vi "Test Conversion.vi"() -> ()   [LabVIEW 2019]
uses:
  src/LV-Data/Typedefs/Map Variant--map.ctl
  <vilib>/numeric/Random Number (Range) U64.vi
  911225dc-c2b6-4d76-ae4e-277c5c34a072.vi
  d4c5f304-fa73-4c90-9b23-d6e558735612.vi
  816afb6b-e639-4658-a948-892f8dd4d78c.vi
  34a72b23-9838-41ec-bdf0-0bcc8987ef23.vi
  b954400e-7329-474c-b3d3-00700c715f51.vi
  6956be5f-2a95-4b1f-9b4a-a21892b67302.vi
  13e05168-3bdc-4092-8862-f966e558d68e.vi
  <vilib>/numeric/sub_Random U32.vi
  <vilib>/Utility/error.llb/Error Cluster From Error Code.vi
  <vilib>/addons/_JKI Toolkits/Caraya/classes/Assert/Assert Not Error.vi
  <vilib>/addons/_JKI Toolkits/Caraya/classes/Assert/Assert Equal Value_Variant.vi
  src/LV-Data/LV-Data.lvclass
  src/LV-Data/Typedefs/Dictionary--cluster.ctl
  67a28817-85e7-4f87-bc92-bf964d179dd8.vi
  8a3b83ae-b8df-4c95-9476-c2011130f52c.vi
  <vilib>/addons/_JKI Toolkits/Caraya/classes/Assert/Assert.lvclass
  <vilib>/addons/_JKI Toolkits/Caraya/classes/Test/Test.lvclass
  1062410e-c2ff-4b72-a76c-15519eba6196.vi
  8f3ef544-03d8-469d-840e-d0608d75c9e5.vi
  e7935e97-479f-40e8-b078-1270a83fd246.vi
  659dfe99-23c1-490f-adb0-d33db7cdd4af.vi
  9b5e4c3a-7fbc-4282-901b-96fdef63c3b4.vi
  ab6de79c-ddce-4639-a401-a316765e1df0.vi
  d3cd4761-c234-4856-afda-8410155b0f64.vi
  24692565-c9bd-4458-b44d-b9188980835d.vi
  fa3941a9-cd6a-4363-9da3-8365bfb5a051.vi
  87514284-9421-4ee1-a24c-5fed3712481b.vi
  src/LV-Data/API/XY-Data to Dictionary (single).vi
  src/LV-Data/API/XY-Data to Dictionary (Multiple).vi
panel:
  in  "Numeric":i32
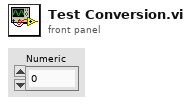
[diagram p1: front panel]
types:
  T1 = typedef "LV-Data.lvclass/Map Variant--map.ctl" = map{string, variant}
  T2 = typedef "LV-Data.lvclass/Dictionary--cluster.ctl" = cluster{"key":string, "value":variant}
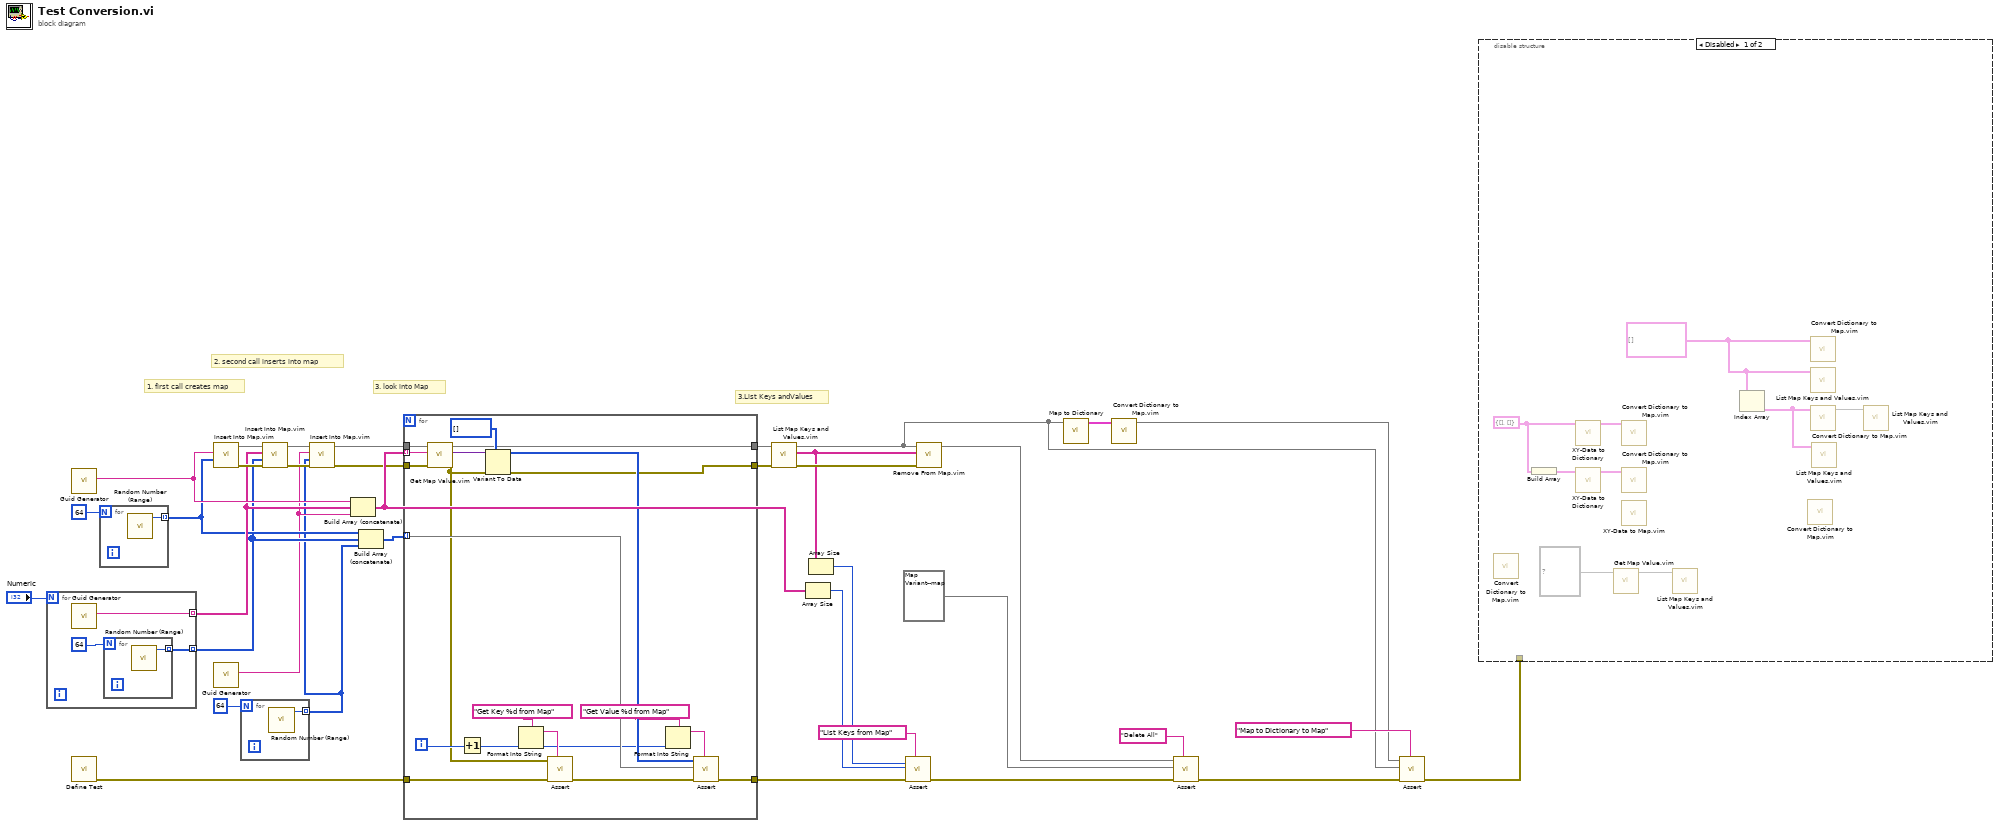
[diagram p0: block diagram]
diagram:
  # "3.List Keys andValues"
  # "3. look into Map"
  # "2. second call inserts into map"
  # "1. first call creates map"
  n1 = for {
    N: "Numeric" -> [_]
    tunnel: [w38] -> w28 mode=indexing
    tunnel: [w37] -> w26 mode=indexing
    n2 = call <vilib>:"Guid Generator.vi"() -> ("GUID"=w38:string)  [unwired: 10 in, 1 out]
    n3 = for {
      N: 64 -> [_]
      tunnel: [w40] -> w37 mode=indexing
      n4 = call-poly <vilib>:"Random Number (Range).vi"() -> ("number"=w40:u64)  [unwired: 11 in]
    }
  }
  n5 = call <vilib>:"Guid Generator.vi"() -> ("GUID"=w29:string)  [unwired: 10 in, 1 out]
  n6 = call <vilib>:"Define Test.vi"() -> ("error out"=w24:errorcluster)  [unwired: 10 in, 1 out]
  n7 = for {
    N: 64 -> [_]
    tunnel: [w41] -> w27 mode=indexing
    n8 = call-poly <vilib>:"Random Number (Range).vi"() -> ("number"=w41:u64)  [unwired: 11 in]
  }
  n9 = call "Insert Into Map.vim"("value"=w27, "key"=w29) -> ("error out"=w30:errorcluster, "map out"=w31:T1)  [unwired: 8 in]
  n10 = call <vilib>:"Guid Generator.vi"() -> ("GUID"=w4:string)  [unwired: 10 in, 1 out]
  n11 = for {
    N: 64 -> [_]
    tunnel: [w42] -> w1 mode=indexing
    n12 = call-poly <vilib>:"Random Number (Range).vi"() -> ("number"=w42:u64)  [unwired: 11 in]
  }
  n13 = call "Insert Into Map.vim"("error in (no error)"=w30, "value"=w26, "key"=w28, "map in"=w31) -> ("error out"=w7:errorcluster, "map out"=w8:T1)  [unwired: 6 in]
  n14 = call "Insert Into Map.vim"("error in (no error)"=w7, "value"=w1, "key"=w4, "map in"=w8) -> ("error out"=w2:errorcluster, "map out"=w3:T1)  [unwired: 6 in]
  n15 = Build Array (concatenate)(w29, w28, w4) -> (w21:string[])
  n16 = Build Array (concatenate)(w27, w26, w1) -> (w25:u64[][])
  n17 = for {
    tunnel: w3 -> [w61]
    tunnel: w21 -> [w60] mode=indexing
    tunnel: w2 -> [w57]
    tunnel: w25 -> [w52] mode=indexing
    tunnel: w24 -> [w51]
    tunnel: [w50] -> w23
    tunnel: [w45] -> w22
    tunnel: [w44] -> w18
    i -> [w47]
    n18 = call "Get Map Value.vim"("error in (no error)"=w57, "Key"=w60, "map in"=w61) -> ("error out"=w46:errorcluster, "value"=w58:variant, "map out"=w45:T1)  [unwired: 6 in]
    n19 = Increment(x=w47) -> (x+1=w43:i32)
    n20 = Variant To Data(error in=w46, type=u64[] [], Variant=w58) -> (data=w53:u64[], error out=w44:errorcluster)
    n21 = Format Into String(format string="Get Key %d from Map" ("Label"), w43) -> (resulting string=w54:string)  [unwired: 2 in, 1 out]
    n22 = call-poly <vilib>:"Assert.vi"("Label"=w54, "error in (no error)"=w51, "Not Error?"=w46) -> ("error out"=w56:errorcluster)  [unwired: 7 in, 1 out]
    n23 = Format Into String(format string="Get Value %d from Map" ("Label"), w43) -> (resulting string=w48:string)  [unwired: 2 in, 1 out]
    n24 = call-poly <vilib>:"Assert.vi"("Label"=w48, "error in (no error)"=w56, "Y"=w52, "X"=w53) -> ("error out"=w50:errorcluster)  [unwired: 6 in, 1 out]
  }
  n25 = call "List Map Keys and Values.vim"("error in (no error)"=w18, "map in"=w22) -> ("error out"=w17:errorcluster, "Keys"=w16:string[], "map out"=w11:T1)  [unwired: 6 in, 1 out]
  n26 = Array Size(array=w21) -> (size(s)=w19:i32)
  n27 = Array Size(array=w16) -> (size(s)=w20:i32)
  n28 = call-poly <vilib>:"Assert.vi"("Label"="List Keys from Map", "error in (no error)"=w23, "Y"=w19, "X"=w20) -> ("error out"=w36:errorcluster)  [unwired: 6 in, 1 out]
  n29 = call "Remove From Map.vim"("error in (no error)"=w17, "key"=w16, "map in"=w11) -> ("map out"=w15:T1)  [unwired: 6 in, 2 out]
  n30 = call "Map to Dictionary.vi"("map"=w11) -> ("Data (Dictionary)"=w13:T2[])  [unwired: 9 in, 1 out]
  n31 = call "Convert Dictionary to Map.vim"("Data (Dictionary)"=w13) -> ("map out"=w12:T1)  [unwired: 9 in, 1 out]
  n32 = call-poly <vilib>:"Assert.vi"("Label"="Delete All", "error in (no error)"=w36, "Y"=T1 {} ("map out"), "X"=w15) -> ("error out"=w10:errorcluster)  [unwired: 6 in, 1 out]
  n33 = call-poly <vilib>:"Assert.vi"("Label"="Map to Dictionary to Map", "error in (no error)"=w10, "Y"=w11, "X"=w12) -> ("error out"=w32:errorcluster)  [unwired: 6 in, 1 out]
  n34 = disable-structure shown="Disabled" {
    disable-tunnel: w32 -> [_ _]
    frame Disabled {
      w62 = cluster{"X-array":dbl[], "Y-array":dbl[]} {"X-array"=[], "Y-array"=[]} ("XY-data in")
      w67 = T2[] [] ("Data")
      n35 = call "Convert Dictionary to Map.vim"() -> ()  [unwired: 10 in, 2 out]
      n36 = Build Array(w62) -> (w65:cluster{"X-array":dbl[], "Y-array":dbl[]}[])
      n37 = call-poly "XY-Data to Dictionary.vi"("XY-data in"=w62) -> ("Data (Dictionary)"=w64:T2[])  [unwired: 9 in, 1 out]
      n38 = call-poly "XY-Data to Dictionary.vi"("XY-data in"=w65) -> ("Data (Dictionary)"=w63:T2[])  [unwired: 9 in, 1 out]
      n39 = call "Get Map Value.vim"("map in"=map{string, variant} {} ("map")) -> ("map out"=w69:map{string, variant})  [unwired: 8 in, 2 out]
      n40 = call "Convert Dictionary to Map.vim"("Data (Dictionary)"=w64) -> ()  [unwired: 9 in, 2 out]
      n41 = call "Convert Dictionary to Map.vim"("Data (Dictionary)"=w63) -> ()  [unwired: 9 in, 2 out]
      n42 = call "XY-Data to Map.vim"() -> ()  [unwired: 10 in, 2 out]
      n43 = call "List Map Keys and Values.vim"("map in"=w69) -> ()  [unwired: 7 in, 4 out]
      n44 = Index Array(array=w67) -> (element=w66:T2)  [unwired: 1 in]
      n45 = call "Convert Dictionary to Map.vim"() -> ()  [unwired: 10 in, 2 out]
      n46 = call "Convert Dictionary to Map.vim"("Data (Dictionary)"=w67) -> ()  [unwired: 9 in, 2 out]
      n47 = call "List Map Keys and Values.vim"("map in"=w67) -> ()  [unwired: 7 in, 4 out]
      n48 = call "Convert Dictionary to Map.vim"("Data (Dictionary)"=w66) -> ("map out"=w68:T1)  [unwired: 9 in, 1 out]
      n49 = call "List Map Keys and Values.vim"("map in"=w66) -> ()  [unwired: 7 in, 4 out]
      n50 = call "List Map Keys and Values.vim"("map in"=w68) -> ()  [unwired: 7 in, 4 out]
    }
    frame Enabled {
    }
  }
